vi "niFpgaZeroCrossingTemplate.vi"(0 "input":fxp<+/-,16,16>, 1 "reset":bool, 7 "direction":enum8{"either", "minus-plus", "plus-minus"}(ring)) -> (4 "crossing":bool)   [LabVIEW 2017]
doc: "Detects zero crossings of an input signal. The data type you wire to <B>input</B> determines the <B>output</B> data type."
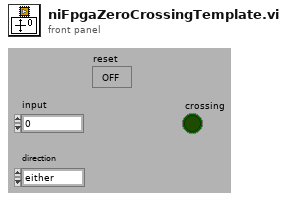
[diagram p1: front panel]
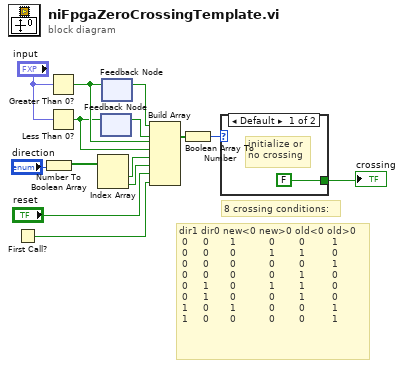
[diagram p0: block diagram]
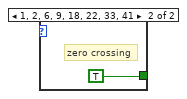
[diagram p2: hidden frame]
diagram:
  # "8 crossing conditions:"
  # "dir1 dir0 new<0 new>0 old<0 old>0\n 0     0       1           0        0         1\n 0     0       0           1        1         0\n 0     0       0           0        0         1\n 0     0       0           0        1         0\n 0     1       0           1        1         0\n 0     1       0           0        1         0\n 1     0       1           0        0         1\n 1     0       0           0        0         1"
  n1 = First Call?() -> (First Call?: T/F=w4:bool)
  n2 = Number To Boolean Array(number="direction") -> (Boolean array=w7:bool[])
  n3 = Greater Than 0?(x="input") -> (x > 0?=w10:bool)
  n4 = Less Than 0?(x="input") -> (x < 0?=w9:bool)
  n5 = Index Array(array=w7) -> (element #1=w6:bool, element #2=w2:bool)  [unwired: 2 in]
  n6 = feedback-in #1(w9) -> ()
  n7 = feedback #1() -> (w11:bool)  [unwired: 1 in]
  n8 = feedback-in #2(w10) -> ()
  n9 = feedback #2() -> (w12:bool)  [unwired: 1 in]
  n10 = Build Array(w12, w11, w10, w9, w6, w2, "reset", w4) -> (w8:bool[])
  n11 = Boolean Array To Number(Boolean array=w8) -> (number=w3:u8)
  n12 = case shown="Default" w3 {
    tunnel: [FALSE TRUE] -> w1
    frame Default {
      # "initialize or\nno crossing"
    }
    frame 1, 2, 6, 9, 18, 22, 33, 41 {
      # "zero crossing"
    }
  }
  "crossing" <- w1
